vi "430_TCP_PSoff.vi"(0 "IP Address":string="111.111.111.2", 2 "TCP Port":i32=7180, 3 "timeout ms (2000)":i32=2000, 5 "error in (no error)":errorcluster, 8 "Switch Heater Control":bool) -> (6 "connection ID":refnum<k5>, 7 "Init Response":string="American Magnetics Model 430 IP Interface\r\nHello.\r\n")   [LabVIEW 2009]
panel:
  out "error out 2":T1
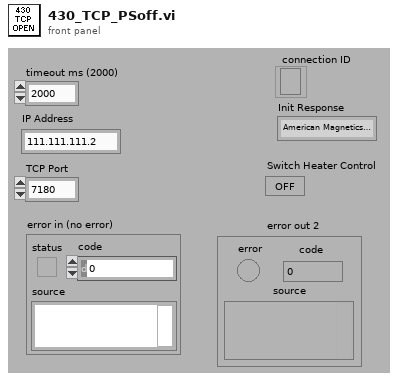
[diagram p1: front panel]
types:
  T1 = cluster{"error":bool, "code":i32, "source":string}
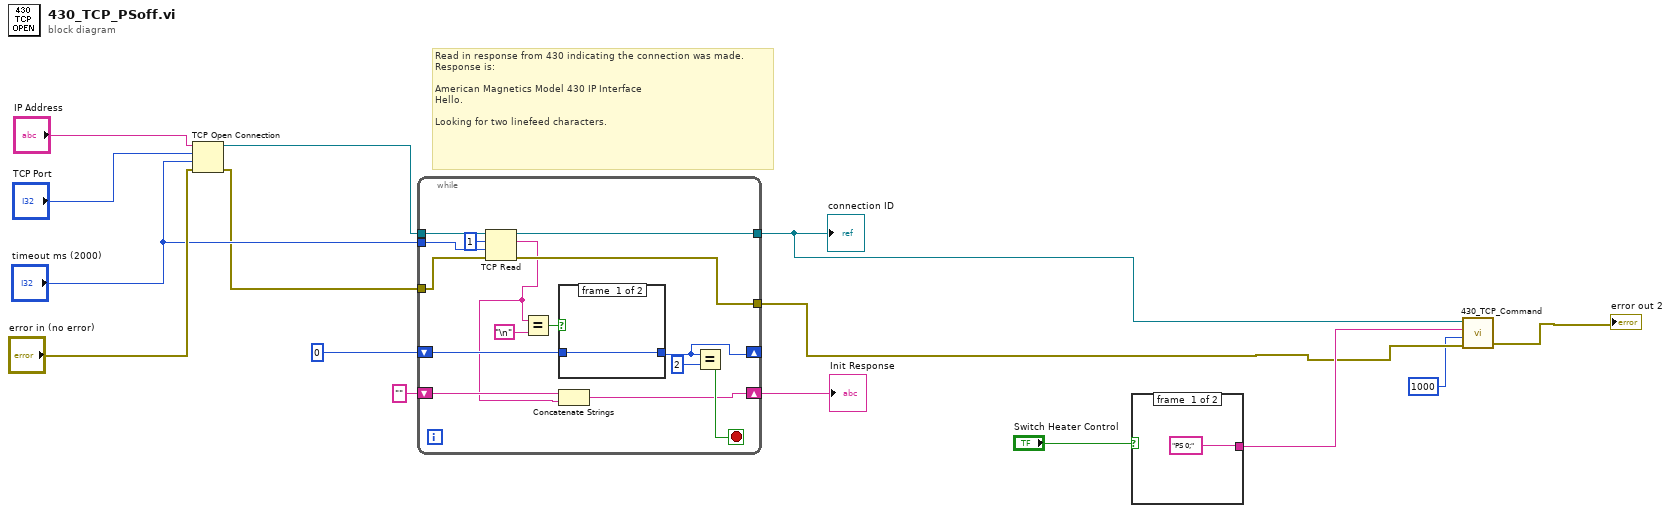
[diagram p0: block diagram]
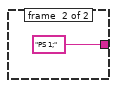
[diagram p2: hidden frame]
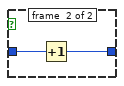
[diagram p3: hidden frame]
diagram:
  # "Read in response from 430 indicating the connection was made.\nResponse is:\n\nAmerican Magnetics Model 430 IP Interface\nHello.\n\nLooking for two linefeed characters."
  n1 = TCP Open Connection(address="IP Address", remote port or service name="TCP Port", timeout ms (60000)="timeout ms (2000)", error in (no error)="error in (no error)") -> (connection ID=w12:refnum<k5>, error out=w9:errorcluster)  [unwired: 1 in]
  n2 = while {
    tunnel: w12 -> [w30]
    tunnel: [w29] -> w3
    tunnel: "timeout ms (2000)" -> [w27]
    tunnel: w9 -> [w26]
    tunnel: [w25] -> w2
    shift-right: [w18] -> w7
    shift-left: "" -> [w19]
    shift-right: [w16] -> _
    shift-left: 0 -> [w24]
    stop <- w22 stop-if-true
    n3 = TCP Read(connection ID=w30, bytes to read=1, error in (no error)=w26, 9:w27) -> (connection ID out=w29:refnum<k5>, data out=w17:string, error out=w25:errorcluster)  [unwired: 1 in]
    n4 = Equal?(x=w17, y="\n") -> (x = y?=w21:bool)
    n5 = case shown="False" w21 {
      tunnel: w24 -> [w31 w33]
      tunnel: [w31 w32] -> w16
      frame #0 {
      }
      frame #1 {
        n6 = Increment(x=w33) -> (x+1=w32:i32)
      }
    }
    n7 = Concatenate Strings(w19, w17) -> (w18:string)
    n8 = Equal?(x=w16, y=2) -> (x = y?=w22:bool)
  }
  "connection ID" <- w3
  "Init Response" <- w7
  n9 = case shown="False" "Switch Heater Control" {
    tunnel: ["PS 0;" "PS 1;"] -> w4
    frame #0 {
    }
    frame #1 {
    }
  }
  n10 = call "430_TCP_Command.vi"("error in (no error)"=w2, "Timeout"=1000, "Command"=w4, "connection ID"=w3) -> ("error out"=→"error out 2":errorcluster)  [unwired: 2 out]
